vi "aim Controller.vi"(8 "error in":errorcluster) -> ()   [LabVIEW 2017]
doc: "This VI executes continuously carrying out the current operation and responding to updates or new operations. It will often contain the timing or control code that is difficult to place directly in TeleOp. This VI generally opens all sensors and motors and isolates the rest of the robot code from knowing how the operations are carried out."
uses:
  <vilib>/Rock Robotics/WPI/Framework/Completion Status.ctl
  aim Setpoints.ctl
  aim Operations.ctl
  <vilib>/Rock Robotics/SystemInterfaces/DIO/FPGA_DIOPWMChannel.ctl
  <vilib>/Rock Robotics/SystemInterfaces/DIO/FPGA_DIOChannel.ctl
  <vilib>/Rock Robotics/WPI/Counter/WPI_CounterDigitalInputToDigitalSource.vi
  <vilib>/Rock Robotics/WPI/Switch/WPI_SwitchOpenLimit.vi
  <vilib>/Rock Robotics/WPI/MotorControl/WPI_MotorControlOpen SPARK.vi
  <vilib>/Rock Robotics/Network Tables/NT Write Boolean.vi
panel:
  in  "Interactive Values":T1
  out "Current\nCmd":string
  in  "Buttons":cluster{"Execute Cmd":bool, "Abort Cmd":bool}
  out "Command Timing":cluster{"Start Time (ms)":u32, "Iterations":i32}
  out "Status":T3
  # "Tip: It may be helpful to observe inputs and sensor values.\nYou may also want to display tuning or debugging controls."
  # "Interactive Command: You may fill in the settings for a command\nand schedule it with the Execute button. You can observe and abort\nany command while fine tuning the code for the controller."
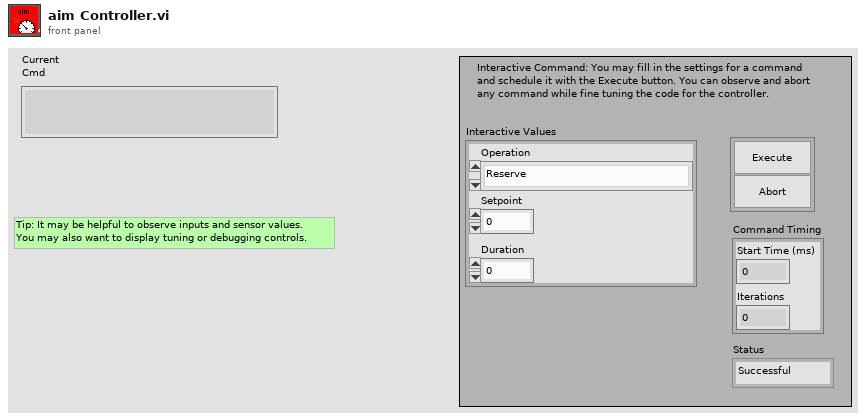
[diagram p1: front panel]
types:
  T1 = typedef "aim Setpoints.ctl" = cluster{"Operation":T2, "Setpoint":dbl, "Duration":dbl}
  T2 = typedef "aim Operations.ctl" = enum16{"Reserve", "Read Current", "Immediate", "position"}
  T3 = typedef "Completion Status.ctl" = enum16{"Successful", "Aborted", "Incomplete"}
  T4 = typedef "FPGA_DIOChannel.ctl" = enum8{"DIO 0", "DIO 1", "DIO 2", "DIO 3", "DIO 4", "DIO 5", "DIO 6", "DIO 7", "DIO 8", "DIO 9", "DIO MXP 0", "DIO MXP 1", "DIO MXP 2", "DIO MXP 3", "DIO MXP 4", "DIO MXP 5", "DIO MXP 6", "DIO MXP 7", "DIO MXP 8", "DIO MXP 9", "DIO MXP 10", "DIO MXP 11", "DIO MXP 12", "DIO MXP 13", "DIO MXP 14", "DIO MXP 15", "SPI Port CS1", "SPI Port CS2", "SPI Port CS3", "SPI Port MISO", "SPI Port MOSI", "Invalid"}
  T5 = typedef "FPGA_DIOPWMChannel.ctl" = enum8{"PWM 0", "PWM 1", "PWM 2", "PWM 3", "PWM 4", "PWM 5", "PWM 6", "PWM 7", "PWM 8", "PWM 9", "PWM MXP 0", "PWM MXP 1", "PWM MXP 2", "PWM MXP 3", "PWM MXP 4", "PWM MXP 5", "PWM MXP 6", "PWM MXP 7", "PWM MXP 8", "PWM MXP 9", "Invalid"}
  T6 = typedef "WPI_SwitchDevRef.ctl" = cluster{"DevStatus":errorcluster, "DIO Channel":T4, "CntIndex":T7, "Normally Closed":bool}
  T7 = typedef "FPGA_CounterCtrSystemIndex.ctl" = enum8{"Ctr 0", "Ctr 1", "Ctr 2", "Ctr 3", "Ctr 4", "Ctr 5", "Ctr 6", "Ctr 7", "Invalid"}
  T8 = typedef "WPI_MotorControlDeviceRef.ctl" = cluster{"DeviceStatus":errorcluster, "Type":T9, "PWM":cluster{"PWM Channel":T5, "DeadBand":T10}, "CAN":cluster{"Device Number":u8, "SetOutput VI Ref":variant, "GetOutput VI Ref":variant, "Enable VI Ref":variant, "Disable VI Ref":variant, "Data":variant}, "Invert":bool, "DIO PWM":cluster{"PWM \"Enable\" Channel":T5, "DIOChannel":T4, "PWM Rate":dbl}}
  T9 = typedef "WPI_MotorControlType.ctl" = enum16{"PWM", "CAN", "DIO PWM"}
  T10 = typedef "WPI_PWMDeadband.ctl" = cluster{"Name":string, "maxPositivePwm":i32, "minPositivePwm":i32, "centerPwm":i32, "maxNegativePwm":i32, "minNegativePwm":i32, "angularRange":u16}
  T11 = typedef "WPI_DigitalInputDevRef.ctl" = cluster{"DevStatus":errorcluster, "DIO Channel":T4}
  T12 = typedef "FPGA_CounterEncoderSourceConvertionLVSourceType.ctl" = cluster{"DevStatus":errorcluster, "AnalogTriggerMode?":bool, "DigitalMode":cluster{"DIO Channel":T13}, "AnalogTriggerMode":cluster{"AnalogTriggerIndex":T14, "OutputType":T15}}
  T13 = typedef "FPGA_DIODigitalSourceChannel.ctl" = enum8{"DIO 0", "DIO 1", "DIO 2", "DIO 3", "DIO 4", "DIO 5", "DIO 6", "DIO 7", "DIO 8", "DIO 9", "DIO MXP 0", "DIO MXP 1", "DIO MXP 2", "DIO MXP 3", "DIO MXP 4", "DIO MXP 5", "DIO MXP 6", "DIO MXP 7", "DIO MXP 8", "DIO MXP 9", "DIO MXP 10", "DIO MXP 11", "DIO MXP 12", "DIO MXP 13", "DIO MXP 14", "DIO MXP 15", "Disabled"}
  T14 = typedef "FPGA_AnalogTriggerIndex.ctl" = enum8{"Trig 0", "Trig 1", "Trig 2", "Trig 3", "Trig 4", "Trig 5", "Trig 6", "Trig 7", "Invalid"}
  T15 = typedef "FPGA_AnalogTriggerOutType.ctl" = enum16{"InWindow", "TriggerState", "Rising", "Falling"}
  T16 = typedef "WPI_EncoderDevRef.ctl" = cluster{"DevStatus":errorcluster, "EncoderIndex":T17, "CounterIndex":T7, "DistancePerCount":dbl, "Decoding Type":T18}
  T17 = typedef "FPGA_EncoderIdx.ctl" = enum8{"Enc 0", "Enc 1", "Enc 2", "Enc 3", "Enc 4", "Enc 5", "Enc 6", "Enc 7", "Invalid"}
  T18 = typedef "WPI_EncoderType.ctl" = enum16{"1x", "2x", "4x"}
  T19 = typedef "Command Status Info.ctl" = cluster{"Name":string, "Status":T3, "notifier out":T20}
  T20 = typedef "Completion Notifier.ctl" = refnum<notifier>
  T21 = cluster{"Current Command":T1, "Command Timing":cluster{"Start Time (ms)":u32, "Iterations":i32}, "Command Arguments":cluster{"Command Info":T19, "Description":string, "Default Command":T1, "queue out":refnum<queue>, "Subsystem Name":string}}
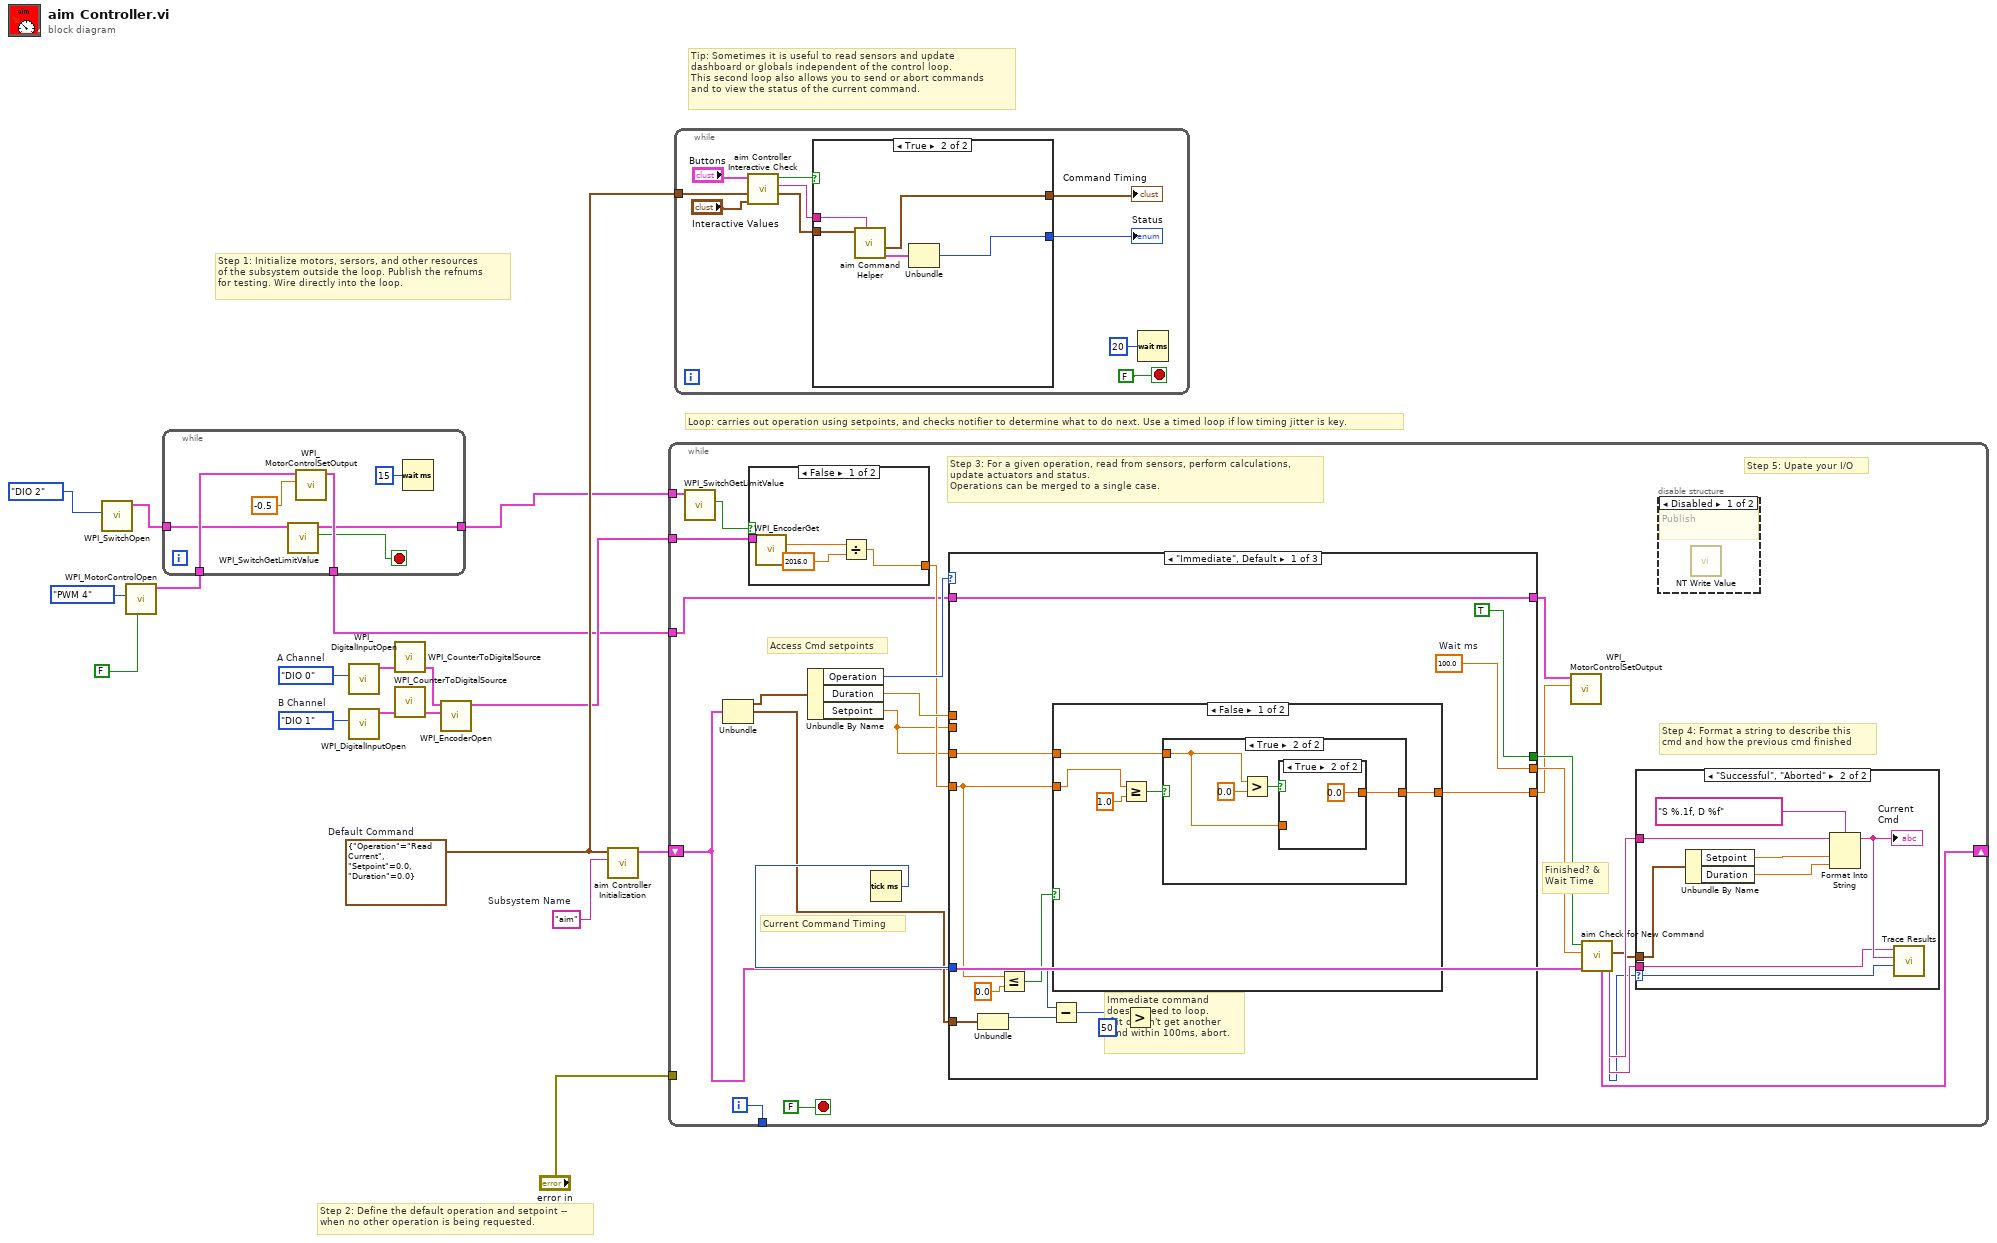
[diagram p0: block diagram]
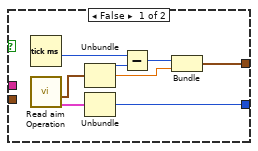
[diagram p2: hidden frame]
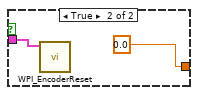
[diagram p3: hidden frame]
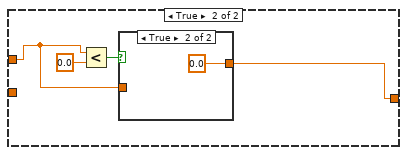
[diagram p8: hidden frame]
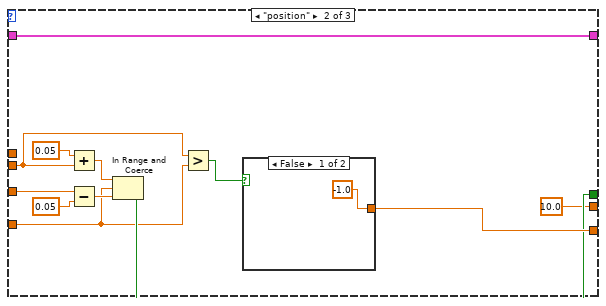
[diagram p10: hidden frame]
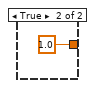
[diagram p11: hidden frame]
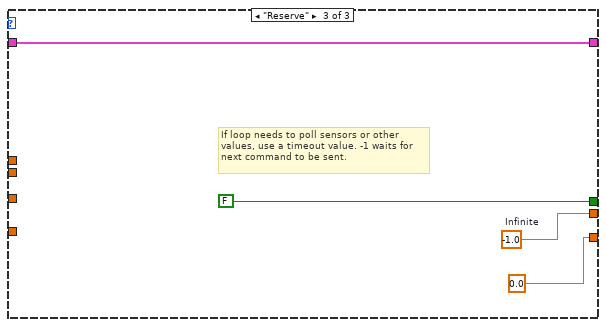
[diagram p12: hidden frame]
diagram:
  w13 = FPGA_DIOChannel."DIO 1"  # B Channel
  w12 = FPGA_DIOChannel."DIO 0"  # A Channel
  w15 = T1 {"Operation"=enum."Read Current", "Setpoint"=0.0, "Duration"=0.0}  # Default Command
  w16 = "aim"  # Subsystem Name
  # "Tip: Sometimes it is useful to read sensors and update\ndashboard or globals independent of the control loop.\nThis second loop also allows you to send or abort commands\nand to view the status of the current command."
  # "Step 2: Define the default operation and setpoint --\nwhen no other operation is being requested."
  # "Step 1: Initialize motors, sersors, and other resources\nof the subsystem outside the loop. Publish the refnums\nfor testing. Wire directly into the loop."
  # "Loop: carries out operation using setpoints, and checks notifier to determine what to do next. Use a timed loop if low timing jitter is key."
  n1 = call-poly <vilib>:"WPI_SwitchOpen.vi"("DIO Channel"=FPGA_DIOChannel."DIO 2") -> ("SwitchDevRef"=w3:T6)  [unwired: 9 in, 1 out]
  n2 = call-poly <vilib>:"WPI_MotorControlOpen.vi"("Invert"=FALSE, "PWM Channel"=FPGA_DIOPWMChannel."PWM 4") -> ("MotorControlDeviceRef"=w5:T8)  [unwired: 8 in, 1 out]
  n3 = while {
    tunnel: w5 -> [w25]
    tunnel: [w24] -> w4
    tunnel: w3 -> [w22]
    tunnel: [w21] -> w2
    stop <- w20 stop-if-true
    n4 = call <vilib>:"WPI_SwitchGetLimitValue.vi"("SwitchDevRef"=w22) -> ("Switch Pressed"=w20:bool, "SwitchDevRef"=w21:T6)  [unwired: 8 in, 1 out]
    n5 = call <vilib>:"WPI_MotorControlSetOutput.vi"("Output"=-0.5, "MotorControlDevRef"=w25) -> ("MotorControlDevRef"=w24:T8)  [unwired: 7 in, 2 out]
    n6 = Wait (ms)(milliseconds to wait=u32 15) -> ()  [unwired: 1 out]
  }
  n7 = call <vilib>:"WPI_DigitalInputOpen.vi"("DIO Channel"=w12) -> ("DigitalInputDevRef"=w9:T11)  [unwired: 1 in, 9 out]
  n8 = call <vilib>:"WPI_DigitalInputOpen.vi"("DIO Channel"=w13) -> ("DigitalInputDevRef"=w10:T11)  [unwired: 1 in, 9 out]
  n9 = call-poly <vilib>:"WPI_CounterToDigitalSource.vi"("DigitalInputDevRef"=w9) -> ("Digital Source"=w8:T12)  [unwired: 6 out]
  n10 = call-poly <vilib>:"WPI_CounterToDigitalSource.vi"("DigitalInputDevRef"=w10) -> ("Digital Source"=w11:T12)  [unwired: 6 out]
  n11 = call <vilib>:"WPI_EncoderOpen.vi"("BSource"=w11, "ASource"=w8) -> ("EncoderDevRef"=w6:T16)  [unwired: 6 in, 3 out]
  n12 = call "aim Controller Initialization.vi"("Subsystem Name"=w16, "Default Command"=w15) -> ("Current Command"=w17:T21)  [unwired: 9 in]
  n13 = while {
    shift-right: [w41] -> _
    shift-left: w17 -> [w34]
    tunnel: [w47] -> _
    tunnel: "error in" -> [_]
    tunnel: w2 -> [w32]
    tunnel: w6 -> [w31]
    tunnel: w4 -> [w29]
    i -> [w47]
    stop <- FALSE stop-if-true
    # "Step 5: Upate your I/O"
    # "Step 4: Format a string to describe this\ncmd and how the previous cmd finished"
    # "Current Command Timing"
    # "Access Cmd setpoints"
    # "Finished? &\nWait Time"
    # "Step 3: For a given operation, read from sensors, perform calculations,\nupdate actuators and status.\nOperations can be merged to a single case."
    n14 = call <vilib>:"WPI_SwitchGetLimitValue.vi"("SwitchDevRef"=w32) -> ("Switch Pressed"=w33:bool)  [unwired: 8 in, 2 out]
    n15 = Unbundle(w34) -> ("Current Command"=w46:T1, "Command Timing"=w42:cluster{"Start Time (ms)":u32, "Iterations":i32})  [unwired: 1 out]
    n16 = case shown="False" w33 {
      tunnel: w31 -> [w52 w54]
      tunnel: [w49 0.0] -> w30
      frame False {
        n17 = call <vilib>:"WPI_EncoderGet.vi"("EncoderDevRef"=w52) -> ("Distance"=w51:dbl)  [unwired: 5 in, 5 out]
        n18 = Divide(x=w51, y=2016.0) -> (x/y=w49:dbl)
      }
      frame True {
        n19 = call <vilib>:"WPI_EncoderReset.vi"("EncoderDevRef"=w54) -> ()  [unwired: 9 in, 2 out]
      }
    }
    n20 = Unbundle By Name(w46) -> ("Operation"=w45:T2, "Duration"=w44:dbl, "Setpoint"=w26:dbl)
    n21 = Tick Count (ms)() -> (millisecond timer value=w43:u32)
    n22 = case shown="\"Immediate\", Default" w45 {
      tunnel: [w75 10.0 ("Infinite") w111] -> w39
      tunnel: [TRUE w99 FALSE ("ignore previous (F)")] -> w40
      tunnel: w42 -> [w71 _ _]
      tunnel: w44 -> [_ _ _]
      tunnel: w43 -> [w70 _ _]
      tunnel: w30 -> [w64 w96 _]
      tunnel: w29 -> [w67 w94 w109]
      tunnel: [w67 w94 w109] -> w28
      tunnel: w26 -> [w63 w103 _]
      tunnel: [w65 w100 0.0] -> w27
      tunnel: w26 -> [_ w97 _]
      frame "Immediate", Default {
        w75 = 100.0  # Wait ms
        # "Immediate command\ndoesn't need to loop.\nIf it doesn't get another\nCmd within 100ms, abort."
        n23 = Unbundle(w71) -> ("Start Time (ms)"=w74:u32)  [unwired: 1 out]
        n24 = Less Or Equal?(x=w64, y=0.0) -> (x <= y?=w69:bool)
        n25 = Subtract(x=w70, y=w74) -> (x-y=w73:u32)
        n26 = case shown="False" w69 {
          tunnel: w64 -> [w77 _]
          tunnel: [w78 w89] -> w65
          tunnel: w63 -> [w76 w88]
          frame False {
            n27 = Greater Or Equal?(x=w77, y=1.0) -> (x >= y?=w79:bool)
            n28 = case shown="True" w79 {
              tunnel: [w81 w83] -> w78
              tunnel: w76 -> [w81 w82]
              frame False {
              }
              frame True {
                n29 = Greater?(x=w82, y=0.0) -> (0:w84:bool)
                n30 = case shown="True" w84 {
                  tunnel: [w86 0.0] -> w83
                  tunnel: w82 -> [w86 _]
                  frame False {
                  }
                  frame True {
                  }
                }
              }
            }
          }
          frame True {
            n31 = Less?(x=w88, y=0.0) -> (x < y?=w90:bool)
            n32 = case shown="True" w90 {
              tunnel: [w92 0.0 ("Output")] -> w89
              tunnel: w88 -> [w92 _]
              frame False {
              }
              frame True {
              }
            }
          }
        }
        n33 = Greater?(x=w73, y=u8 50 ("Left Motor")) -> ()  [unwired: 1 out]
      }
      frame "position" {
        n34 = Add(x=0.05 ("Duration"), y=w97) -> (x+y=w101:dbl)
        n35 = Subtract(x=w103, y=0.05 ("Setpoint")) -> (x-y=w102:dbl)
        n36 = In Range and Coerce(upper limit=w101, x=w96, lower limit=w102) -> (In Range?=w99:bool)  [unwired: 1 out]
        n37 = Greater?(x=w97, y=w96) -> (0:w98:bool)
        n38 = case shown="False" w98 {
          tunnel: [-1.0 1.0] -> w100
          frame False {
          }
          frame True {
          }
        }
      }
      frame "Reserve" {
        w111 = -1.0  # Infinite
        # "If loop needs to poll sensors or other\nvalues, use a timeout value. -1 waits for\nnext command to be sent."
      }
    }
    n39 = call <vilib>:"WPI_MotorControlSetOutput.vi"("Output"=w27, "MotorControlDevRef"=w28) -> ()  [unwired: 7 in, 3 out]
    n40 = call "aim Check for New Command.vi"("Current Command"=w34, "Wait time (ms)"=w39, "Finished?"=w40) -> ("Completion"=w35:T3, "Subsystem Name"=w36:string, "Current Command"=w37:T1, "Initial Trace String"=w38:string, "NextCommand"=w41:T21)  [unwired: 4 in]
    n41 = case shown="\"Successful\", \"Aborted\"" w35 {
      selector: w35 -> [_ w62]
      tunnel: w38 -> [_ w58]
      tunnel: w37 -> [_ w59]
      tunnel: w36 -> [_ w55]
      frame "Incomplete", Default {
        # "Continuing current command"
      }
      frame "Successful", "Aborted" {
        # "Report and setup for next command"
        n42 = Unbundle By Name(w59) -> ("Setpoint"=w61:dbl, "Duration"=w56:dbl)
        n43 = Format Into String(format string="S %.1f, D %f", initial string=w58, w61, w56) -> (resulting string=w57:string)  [unwired: 1 in, 1 out]
        "Current\nCmd" <- w57
        n44 = call <vilib>:"Trace Results.vi"("Status of previous command"=w62, "Description"=w57, "Subsystem"=w55) -> ()  [unwired: 9 in]
      }
    }
    n45 = disable-structure shown="Disabled" {
      frame Disabled {
        # "Publish"
        n46 = call-poly <vilib>:"NT Write Value.vi"() -> ()  [unwired: 11 in, 1 out]
      }
      frame Enabled {
      }
    }
  }
  n47 = while {
    tunnel: w15 -> [w118]
    stop <- FALSE stop-if-true
    n48 = call "aim Controller Interactive Check.vi"("Interactive Command in"="Interactive Values", "Default Command"=w118, "Buttons"="Buttons") -> ("Interactive Command out"=w115:T1, "Trace String"=w116:string, "Schedule"=w117:bool)  [unwired: 6 in]
    n49 = case shown="True" w117 {
      tunnel: [w129 w134] -> w114
      tunnel: w115 -> [_ w132]
      tunnel: [w125 w130] -> w113
      tunnel: w116 -> [_ w133]
      frame False {
        n50 = Tick Count (ms)() -> (millisecond timer value=w124:u32)
        n51 = call "Read aim Operation.vi"() -> ("Command Info"=w122:T19, "SubSystem Data"=w123:T1)  [unwired: 9 in, 1 out]
        n52 = Unbundle(w123) -> ("Operation"=w128:T2, "Setpoint"=w126:dbl)  [unwired: 1 out]
        n53 = Unbundle(w122) -> ("Status"=w129:T3)  [unwired: 2 out]
        n54 = Subtract(x=w124, y=w128) -> (x-y=w127:u32)
        n55 = Bundle(w127, "Setpoint"=w126) -> (w125:cluster{u32, "Setpoint":dbl})  [unwired: 1 in]
      }
      frame True {
        n56 = call "aim Command Helper.vi"("Description"=w133, "SubSystem Data"=w132) -> ("Command Info Out"=w131:T19, "Command Timing"=w130:cluster{"Start Time (ms)":u32, "Iterations":i32})  [unwired: 7 in, 1 out]
        n57 = Unbundle(w131) -> ("Status"=w134:T3)  [unwired: 2 out]
      }
    }
    "Status" <- w114
    "Command Timing" <- w113
    n58 = Wait (ms)(milliseconds to wait=u32 20) -> ()  [unwired: 1 out]
  }
